vi "FdxCmdBITETransferCvi.vi"(8 "error in":errorcluster, 10 "SrvName":string, 11 "Board_ResourceID":u32) -> (0 "error out":errorcluster, 3 "Board_ResourceID Out":u32)   [LabVIEW 2020, in "AIM664LV.lvlib"]
doc: "This function performs some transfer tests using available port resources of one FDX board. This function will determine the number of ports on the board. If only two ports, it will test them against each other. If four ports are used, Port 1 and Port 2 will be tested against each other and Port 3 and Port 4 will be tested against each other. \nPort 1 and Port 2 must be connected with a Loop-Back cable (crossover), if available Port 3 and Port 4 must be connected with a Loop-Back cable (crossover).\nThe resources of the board under test shall be not logged in."
uses:
  AIM664LV.lvlib
  AFDX_LibraryAdmin/FdxGlobalDllPath.vi
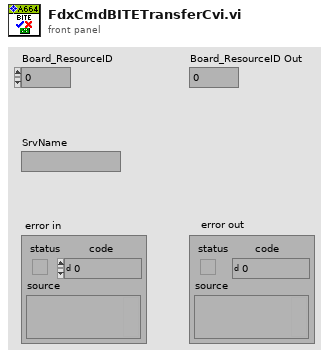
[diagram p1: front panel]
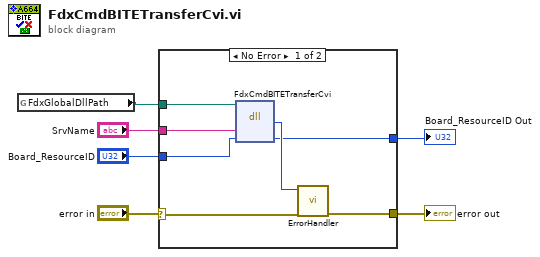
[diagram p0: block diagram]
diagram:
  n1 = global read "FdxGlobalDllPath.vi" "FdxGlobalDllPath"() -> (w4:path)
  n2 = case shown="No Error" "error in" {
    selector: "error in" -> [w12 w15]
    tunnel: [w13 w15] -> w6
    tunnel: w4 -> [w10 _]
    tunnel: "SrvName" -> [w9 _]
    tunnel: "Board_ResourceID" -> [w8 w14]
    tunnel: [w7 w14] -> w1
    frame No Error {
      n3 = dll-call lib="aim_fdx.19.dll" fn="FdxCmdBITETransferCvi"(path in=w10, "SrvName"=w9, "Board_ResourceID"=w8) -> ("status"=w11:i32, "Board_ResourceID"=w7:u32)  [unwired: 2 in, 3 out]
      n4 = call "ErrorHandler.vi"("error in"=w12, "AIM Error"=w11) -> ("error out"=w13:errorcluster)  [unwired: 9 in]
    }
    frame Error {
    }
  }
  "error out" <- w6
  "Board_ResourceID Out" <- w1
